vi "id.vi"(8 "error in (no error)":errorcluster, 11 "TestCase in":refnum<class "TestCase.lvclass">) -> (0 "error out":errorcluster, 1 "GUID":string, 2 "id":string, 3 "TestCase out":refnum<class "TestCase.lvclass">)   [LabVIEW 2011, in "TestCase.lvclass"]
uses:
  TestCase.lvclass
  TestCase.lvclass/TestCase.ctl
  Libraries/VITesterUtilities.lvlib
panel:
  # "JKI VI Tester for LabVIEW\nhttp://jkisoft.com/vi-tester\nCopyright (C) 2007-2009, JKI <info@jkisoft.com>\nALL RIGHTS RESERVED"
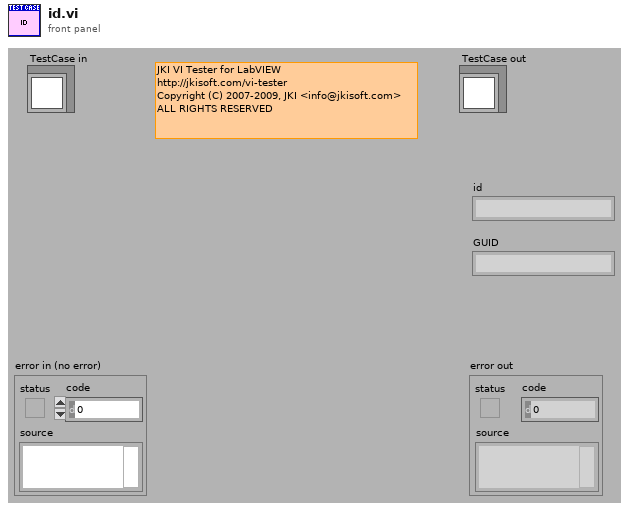
[diagram p1: front panel]
types:
  T1 = typedef "TestCase.lvclass/testMethodName.ctl" = string
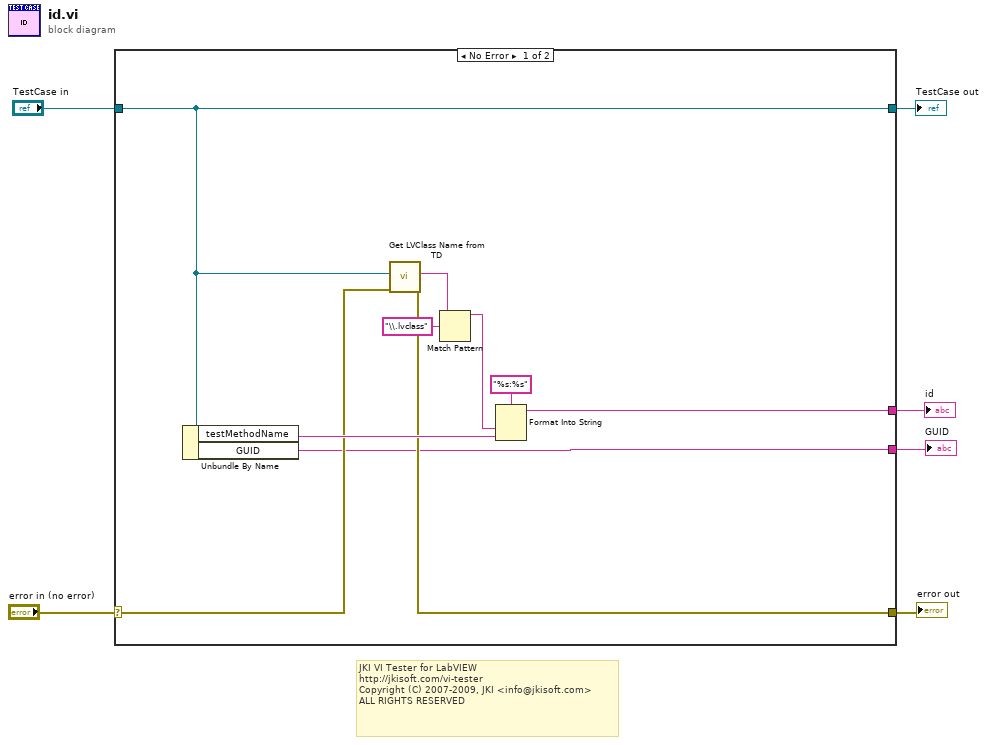
[diagram p0: block diagram]
diagram:
  # "JKI VI Tester for LabVIEW\nhttp://jkisoft.com/vi-tester\nCopyright (C) 2007-2009, JKI <info@jkisoft.com>\nALL RIGHTS RESERVED"
  n1 = case shown="No Error" "error in (no error)" {
    selector: "error in (no error)" -> [w8 w18]
    tunnel: [w14 w18] -> w5
    tunnel: [w9 w17] -> w3
    tunnel: "TestCase in" -> [w9 w17]
    tunnel: [w13 _] -> w2
    tunnel: [w7 _] -> w1
    frame No Error {
      n2 = Unbundle By Name(w9) -> ("testMethodName"=w15:T1, "GUID"=w7:string)
      n3 = call "Get LVClass Name from TD.vi"("error in"=w8, "Variant"=w9) -> ("error out"=w14:errorcluster, "LVClass Name"=w11:string)  [unwired: 8 in]
      n4 = Match Pattern(string=w11, regular expression="\\.lvclass") -> (before substring=w10:string)  [unwired: 1 in, 3 out]
      n5 = Format Into String(format string="%s:%s", w10, w15) -> (resulting string=w13:string)  [unwired: 2 in, 1 out]
    }
    frame Error {
    }
  }
  "error out" <- w5
  "TestCase out" <- w3
  "id" <- w2
  "GUID" <- w1
